vi "set_backlash_option_by_name.vi"(8 "error in (no error)":errorcluster caption="错误输入（无错误）", 9 "backlash option":T1, 10 "name":string, 11 "MotorSystem输入":refnum<class "MotorSystem.lvclass">) -> (0 "error out":errorcluster caption="错误输出", 3 "MotorSystem输出":refnum<class "MotorSystem.lvclass">)   [LabVIEW 2016, in "MotionControl_UFO_3DOF.lvlib" / "MotorSystem.lvclass"]
uses:
  <userlib>/MotionControl_UFO_3DOF/MotorSystem/MotorSystem.lvclass
  <userlib>/MotionControl_UFO_3DOF/OneMotion/backlash option.ctl
  <userlib>/MotionControl_UFO_3DOF/MotorSystem/MotorSystem.lvclass/MotorSystem.ctl
  <userlib>/MotionControl_UFO_3DOF/OneMotion/OneMotion.lvclass/OneMotion.ctl
  <userlib>/MotionControl_UFO_3DOF/OneMotion/OneMotion.lvclass
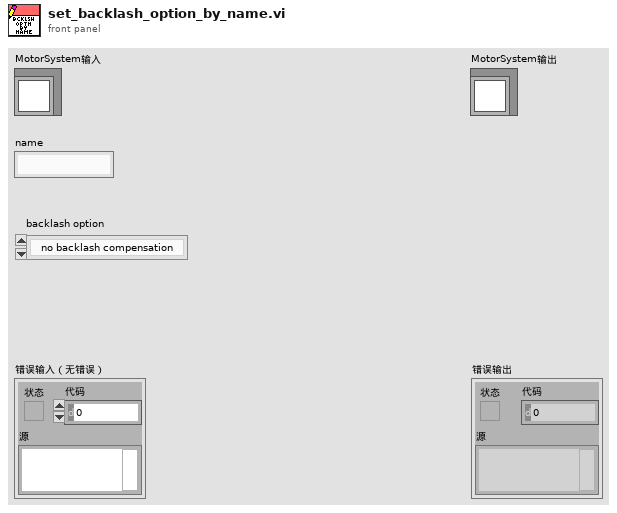
[diagram p1: front panel]
types:
  T1 = typedef "MotionControl_UFO_3DOF.lvlib/OneMotion.lvclass/backlash option.ctl" = enum16{"no backlash compensation", "compensation: from - to +", "compensation: from + to -"}
  T2 = typedef "MotionControl_UFO_3DOF.lvlib/MotorSystem.lvclass/MotionCluster.ctl" = cluster{"OneMotion.lvclass":refnum<class "OneMotion.lvclass">, "connected?":bool, "default enabled?":bool, "enabled?":bool}
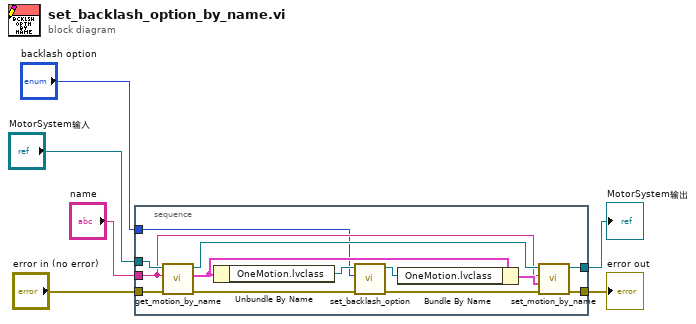
[diagram p0: block diagram]
diagram:
  n1 = stacked-sequence {
    tunnel: [w12] -> w6
    tunnel: [w14] -> w4
    tunnel: "MotorSystem输入" -> [w19]
    tunnel: "name" -> [w15]
    tunnel: "error in (no error)" -> [w13]
    tunnel: "backlash option" -> [w7]
    frame #0 {
      n2 = call <userlib>:"get_motion_by_name.vi"("error in (no error)"=w13, "name"=w15, "MotorSystem in"=w19) -> ("error out"=w11:errorcluster, "motion cluster"=w18:T2, "MotorSystem out"=w17:refnum<class "MotorSystem.lvclass">)  [unwired: 6 in]
      n3 = Unbundle By Name(w18) -> ("OneMotion.lvclass"=w10:refnum<class "OneMotion.lvclass">)
      n4 = call <userlib>:"set_backlash_option.vi"("error in (no error)"=w11, "backlash option"=w7, "OneMotion输入"=w10) -> ("error out"=w8:errorcluster, "OneMotion输出"=w9:refnum<class "OneMotion.lvclass">)  [unwired: 7 in]
      n5 = Bundle By Name(cluster=w18, "OneMotion.lvclass"=w9) -> (w16:T2)
      n6 = call <userlib>:"set_motion_by_name.vi"("error in (no error)"=w8, "簇"=w16, "name"=w15, "MotorSystem输入"=w17) -> ("error out"=w12:errorcluster, "MotorSystem输出"=w14:refnum<class "MotorSystem.lvclass">)  [unwired: 6 in]
    }
  }
  "error out" <- w6
  "MotorSystem输出" <- w4
